vi "ControlMainGUIWindow.vi"(8 "ErrorIn":errorcluster, 10 "ShowProcessWindow":bool, 11 "ReferenceIn":refnum<class "BusBase.lvclass">) -> (0 "ErrorOut":errorcluster, 2 "Dummy":bool, 3 "ReferenceOut":refnum<class "BusBase.lvclass">)   [LabVIEW 2021, in "BusBase.lvlib" / "BusBase.lvclass"]
uses:
  BusBase.lvclass
  protected/BusBase_MessageData.ctl
  9f903c85-2847-4db9-ba05-d8e85b2316fc.vi
  protected/MainGUIRepository.vi
  BusBase.lvclass/BusBase.ctl
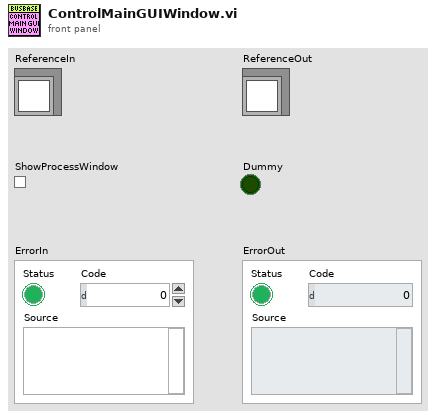
[diagram p1: front panel]
types:
  T1 = typedef "BusBase.lvlib/BusBase.lvclass/BusBase_MessageData.ctl" = cluster{"ShowWindow":cluster{"Send":cluster{"Show":bool}, "Receive":cluster{"Dummy":bool}}}
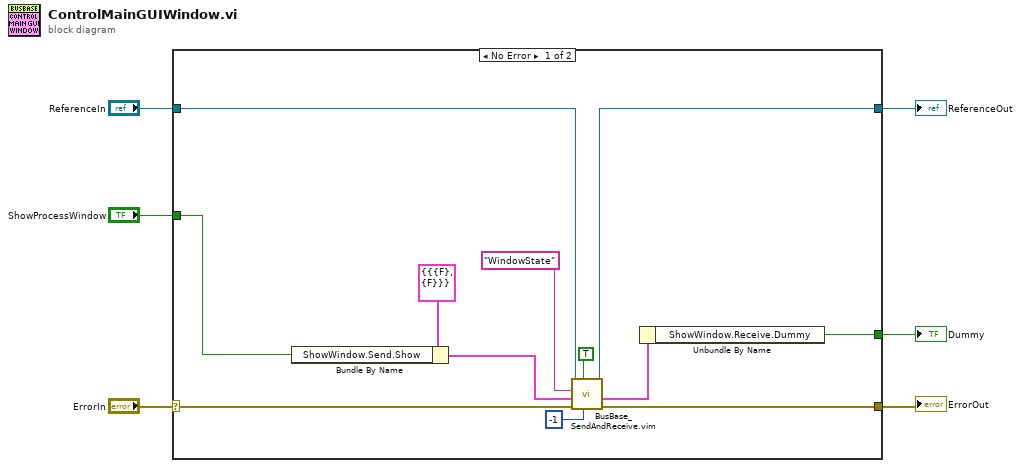
[diagram p0: block diagram]
diagram:
  n1 = case shown="No Error" "ErrorIn" {
    selector: "ErrorIn" -> [w18 w20]
    tunnel: [w17 w20] -> w5
    tunnel: [w14 w19] -> w3
    tunnel: "ReferenceIn" -> [w15 w19]
    tunnel: "ShowProcessWindow" -> [w12 _]
    tunnel: [w9 _] -> w1
    frame No Error {
      n2 = Bundle By Name(cluster=T1 {"ShowWindow"={"Send"={"Show"=FALSE}, "Receive"={"Dummy"=FALSE}}} ("MessageData"), "ShowWindow.Send.Show"=w12) -> (w11:T1)
      n3 = call "BusBase_SendAndReceive.vim"("TimeoutInMs(-1)"=-1 ("timeout in ms (-1)"), "ShouldWeWaitForResponse"=TRUE, "ErrorIn"=w18, "Data"=w11, "Command"="WindowState", "ReferenceIn"=w15) -> ("ErrorOut"=w17:errorcluster, "ReplyData"=w10:T1, "ReferenceOut"=w14:refnum<class "BusBase.lvclass">)  [unwired: 3 in]
      n4 = Unbundle By Name(w10) -> ("ShowWindow.Receive.Dummy"=w9:bool)
    }
    frame Error {
    }
  }
  "ErrorOut" <- w5
  "ReferenceOut" <- w3
  "Dummy" <- w1
